vi "Test_Create_Greyscale.vi"(8 "error in (no error)":errorcluster, 11 "Test Case In":refnum<class "Image.lvclass">) -> (0 "error out":errorcluster, 3 "Test Case Out":refnum<class "Image.lvclass">)   [LabVIEW 2020, in "g_ar_toolkit.test.lvlib" / "Image.lvclass"]
uses:
  Image.lvclass
  Image.lvclass/Image.ctl
  g_ar_toolkit.image/g_ar_toolkit.image.lvlib
  g_ar_toolkit.image/Image Size (Fixed).ctl
  g_ar_toolkit.image/CreateEmptyImageGreyscale.vi
  4993e8ee-a06a-463a-9684-69129f64d5ce.vi
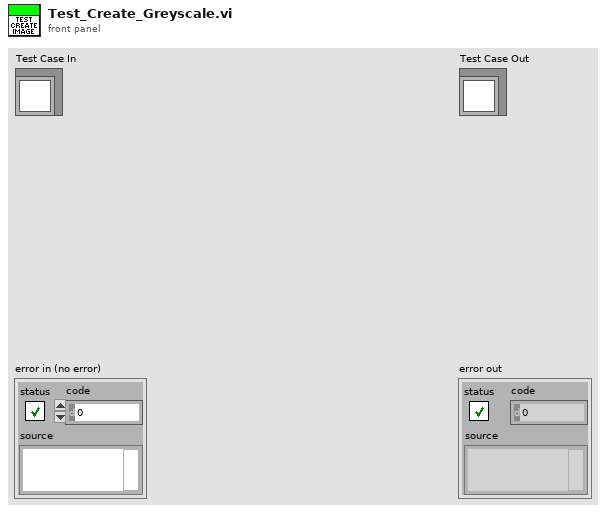
[diagram p1: front panel]
types:
  T1 = typedef "g_ar_toolkit.image.lvlib/Image Size (Fixed).ctl" = cluster{"Width":u16, "Height":u16}
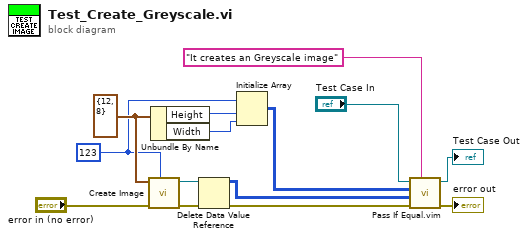
[diagram p0: block diagram]
diagram:
  w3 = u8 123 ("Value (Default: 0)")
  w6 = T1 {"Width"=12, "Height"=8} ("Preallocated Image Size (Default - 0,0)")
  n1 = call-poly "Create Image.vi"("Value (Default: 0)"=w3, "error in (no error)"="error in (no error)", "Preallocated Image Size (Default 0,0)"=w6) -> ("error out"=w9:errorcluster, "New Greyscale Image"=w10:refnum<data-value>)  [unwired: 7 in]
  n2 = Unbundle By Name(w6) -> ("Height"=w5:u16, "Width"=w4:u16)
  n3 = Delete Data Value Reference(data value reference=w10, error in=w9) -> (data value=w1:u8[][], error out=w8:errorcluster)
  n4 = Initialize Array(w3, w5, w4) -> (w2:u8[][])
  n5 = call "Pass If Equal.vim"("Description"="It creates an Greyscale image", "error in (no error)"=w8, "Actual"=w1, "Expected"=w2, "LUnit Test Case In"="Test Case In") -> ("error out"=→"error out":errorcluster, "LUnit Test Case Out"=→"Test Case Out":refnum<class "Image.lvclass">)  [unwired: 5 in]
